vi "LV2_1.vi"() -> ()   [LabVIEW 2011]
uses:
  <vilib>/imath/engines/lvmath2/RunTimeEngine/ErrorHandling/NIMS_Finalize Error.vi
  <vilib>/imath/engines/lvmath2/RunTimeEngine/NodeEndStatement/NIMS_NodeEndStatement_Output.vi
  <instcachedir>/0/NIMS_NodeEndStatement_Output_53EC0D466D134D7ABD903AC30B43404B.lvgen/NIMS_NodeEndStatement_Output_53EC0D466D134D7ABD903AC30B43404B_005.vi
  <vilib>/imath/engines/lvmath2/RunTimeEngine/RangeToken/NIMS_Range.vi
  <instcachedir>/0/NIMS_Range_0B7635FB69F84E19AA68E7FF959DF37C.lvgen/NIMS_Range_0B7635FB69F84E19AA68E7FF959DF37C_001.vi
  <vilib>/imathl/engines/lvmath/Functions/Error Handling/Create Error.vi
  <vilib>/imath/engines/lvmath2/RunTimeEngine/BuiltInFunctions/conv/NIMS_conv(V,V).vi
  <instcachedir>/0/NIMS_conv(V,V)_D3E194F2B5174935BB2368CEB7AAC5A9.lvgen/NIMS_conv(V,V)_D3E194F2B5174935BB2368CEB7AAC5A9_000.vi
  <vilib>/imath/engines/lvmath2/RunTimeEngine/ErrorHandling/NIMS_Error From Error Code.vi
  <vilib>/imath/engines/lvmath2/RunTimeEngine/ArithmeticOperatorToken/NIMS_ArithmeticOperator_minus.vi
  <instcachedir>/0/NIMS_ArithmeticOperator_minus_27860A2576AF4B729B9D72749D8AAD88.lvgen/NIMS_ArithmeticOperator_minus_27860A2576AF4B729B9D72749D8AAD88_003.vi
panel:
  out "Convolution (numeric)":cluster{"TY":dbl[], "Y":dbl[]}(graph)
  in  "Stop Button":bool
  in  "decay2":dbl(slide) scale=1.0..10.0
  in  "decay1":dbl(slide) scale=1.0..10.0
  out "Signals":cluster{"T":dbl[], "X":dbl[]}[](graph)
  out "Convolution (analytic)":cluster{"TY":dbl[], "YACT":dbl[]}(graph)
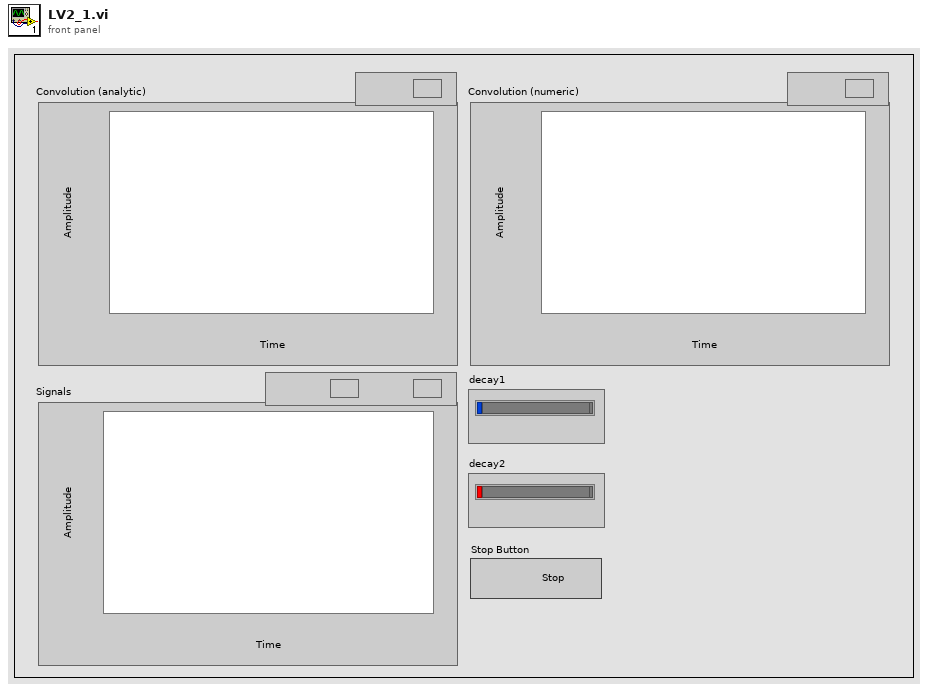
[diagram p1: front panel]
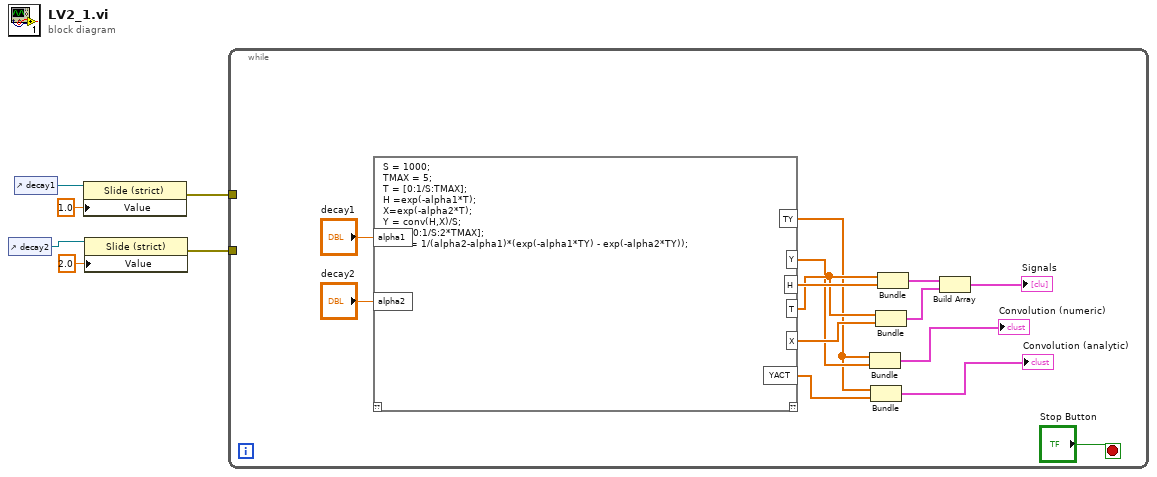
[diagram p0: block diagram]
diagram:
  n1 = control-ref of="decay2"() -> (w2:refnum<vi>)
  n2 = control-ref of="decay1"() -> (w6:refnum<vi>)
  n3 = property class="Slide (strict)"(reference=w6, "Value"=1.0) -> (error out=w5:errorcluster)  [unwired: 1 in, 1 out]
  n4 = property class="Slide (strict)"(reference=w2, "Value"=2.0) -> (error out=w1:errorcluster)  [unwired: 1 in, 1 out]
  n5 = while {
    tunnel: w5 -> [_]
    tunnel: w1 -> [_]
    stop <- "Stop Button" stop-if-true
    n6 = mathscript code="S = 1000;\nTMAX = 5;\nT = [0:1/S:TMAX];\nH =exp(-alpha1*T);\nX=exp(-alpha2*T);\nY = conv(H,X)/S;\nTY = [0:1/S:2*TMAX];\nYACT = 1/(alpha2-alpha1)*(exp(-alpha1*TY) - exp(-alpha2*TY));"("alpha1"="decay1", "alpha2"="decay2") -> ("TY"=w14:dbl[], "Y"=w15:dbl[], "H"=w20:dbl[], "X"=w18:dbl[], "YACT"=w13:dbl[], "T"=w19:dbl[])  [unwired: 1 in, 1 out]
    n7 = Bundle("TY"=w14, "Y"=w15) -> (→"Convolution (numeric)":cluster{"TY":dbl[], "Y":dbl[]})  [unwired: 1 in]
    n8 = Bundle("TY"=w14, "YACT"=w13) -> (→"Convolution (analytic)":cluster{"TY":dbl[], "YACT":dbl[]})  [unwired: 1 in]
    n9 = Bundle("T"=w19, "X"=w18) -> (w16:cluster{"T":dbl[], "X":dbl[]})  [unwired: 1 in]
    n10 = Bundle("T"=w19, "H"=w20) -> (w17:cluster{"T":dbl[], "H":dbl[]})  [unwired: 1 in]
    n11 = Build Array(w17, w16) -> (→"Signals":cluster{"T":dbl[], "X":dbl[]}[])
  }
